vi "Login.vi"(8 "Error In":errorcluster, 10 "UserInfo":cluster{"User":string, "Value":string}, 11 "menu reference":refnum<k9>) -> (0 "Error Out":errorcluster)   [LabVIEW 2025, in "Full User Interface.lvlib"]
uses:
  Full User Interface.lvlib
  Localization/Section.ctl
  Localization/Localization.lvlib
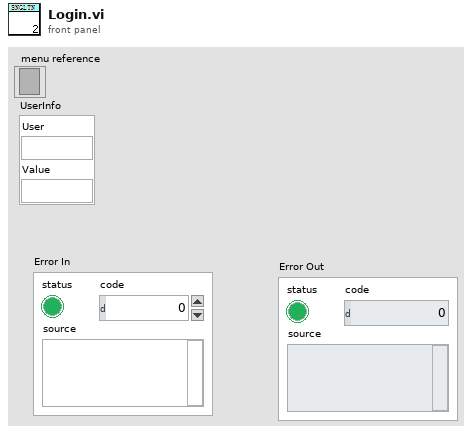
[diagram p1: front panel]
types:
  T1 = typedef "Localization.lvlib/Section.ctl" = enum16{"Menu", "Title", "Workstation Config"}
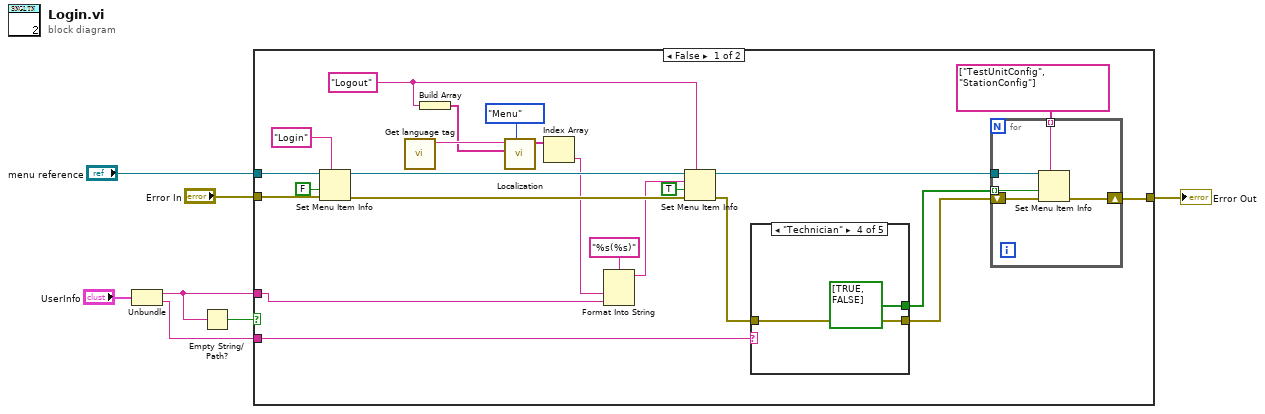
[diagram p0: block diagram]
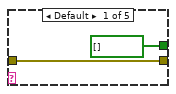
[diagram p2: hidden frame]
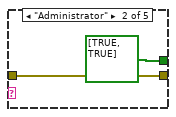
[diagram p3: hidden frame]
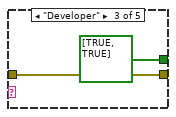
[diagram p4: hidden frame]
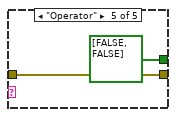
[diagram p5: hidden frame]
diagram:
  n1 = Unbundle("UserInfo") -> ("User"=w4:string, "Value"=w1:string)
  n2 = Empty String/Path?(string/path=w4) -> (empty?=w5:bool)
  n3 = case shown="False" w5 {
    tunnel: "menu reference" -> [w30 _]
    tunnel: w4 -> [w9 _]
    tunnel: [w18 w46] -> w3
    tunnel: "Error In" -> [w23 w46]
    tunnel: w1 -> [w21 _]
    frame False {
      w10 = "Logout"
      n4 = Set Menu Item Info(7:"Login", 8:w23, 9:FALSE ("enabled"), 11:w30) -> (0:w27:errorcluster, 3:w28:refnum<k9>)  [unwired: 3 in]
      n5 = call "Get language tag.vi"() -> ("language tag"=w13:string)  [unwired: 11 in]
      n6 = Build Array(w10) -> (w12:string[])
      n7 = call "Localization.vi"("section"=Section."Menu", "key"=w12, "Language key"=w13) -> ("Value"=w11:string[])  [unwired: 7 in, 1 out]
      n8 = Index Array(array=w11) -> (element=w8:string)  [unwired: 1 in]
      n9 = Format Into String(format string="%s(%s)", w8, w9) -> (resulting string=w24:string)  [unwired: 2 in, 1 out]
      n10 = Set Menu Item Info(7:w10, 8:w27, 9:TRUE ("enabled"), 10:w24, 11:w28) -> (0:w20:errorcluster, 3:w15:refnum<k9>)  [unwired: 2 in]
      n11 = case shown="\"Technician\"" w21 {
        tunnel: w20 -> [w37 w39 w41 w43 w45]
        tunnel: [w37 w39 w41 w43 w45] -> w19
        tunnel: [bool[] [] bool[] [TRUE, TRUE] bool[] [TRUE, TRUE] bool[] [TRUE, FALSE] bool[] [FALSE, FALSE]] -> w16
        frame Default {
        }
        frame "Administrator" {
        }
        frame "Developer" {
        }
        frame "Technician" {
        }
        frame "Operator" {
        }
      }
      n12 = for {
        shift-right: [w34] -> w18
        shift-left: w19 -> [w35]
        tunnel: string[] ["TestUnitConfig", "StationConfig"] ("item tags") -> [w33] mode=indexing
        tunnel: w16 -> [w32] mode=indexing
        tunnel: w15 -> [w31]
        n13 = Set Menu Item Info(7:w33, 8:w35, 9:w32, 11:w31) -> (0:w34:errorcluster)  [unwired: 3 in, 1 out]
      }
    }
    frame True {
    }
  }
  "Error Out" <- w3
